vi "Close Library.vi"(8 "error in":errorcluster, 11 "Library Icon Data in":refnum<class "Library Icon Data.lvclass">) -> (0 "error out":errorcluster, 3 "Library Icon Data out":refnum<class "Library Icon Data.lvclass">)   [LabVIEW 2020, in "Library Icon Data.lvclass"]
doc: "Closes the Application and Library references."
uses:
  Library Icon Data.lvclass
  Library Icon Data.lvclass/Library Icon Data.ctl
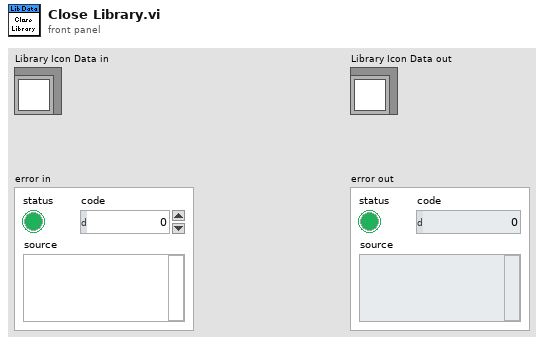
[diagram p1: front panel]
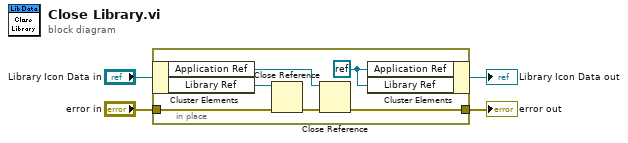
[diagram p0: block diagram]
diagram:
  n1 = in-place {
    in-place-border: "error in" -> [w10]
    in-place-border: [w8] -> w3
    w5 = refnum<k0> refnum
    n2 = in-place-cluster #1("Library Icon Data in") -> ("Application Ref"=w6:refnum<vi>, "Library Ref"=w7:refnum<vi>)
    n3 = Close Reference(reference=w7, error in (no error)=w10) -> (error out=w9:errorcluster)
    n4 = Close Reference(reference=w6, error in (no error)=w9) -> (error out=w8:errorcluster)
    n5 = in-place-cluster #1("Application Ref"=w5, "Library Ref"=w5) -> (→"Library Icon Data out":refnum<class "Library Icon Data.lvclass">)
  }
  "error out" <- w3
